vi "8step.vi"(6 "LINX Resource in":T1, 7 "Angle in":i32, 8 "error in (no error)":errorcluster, 9 "DO Channels":u8[](array[numeric]), 10 "CCW":bool, 11 "OK Button":bool) -> (0 "error out":errorcluster, 2 "LINX Resource out":T1, 3 "Actual angle out":dbl)   [LabVIEW 2020]
uses:
  <vilib>/MakerHub/LINX/Private/Type Defs/LINX Ref.ctl
  <vilib>/MakerHub/LINX/Private/Type Defs/Platform.ctl
  <vilib>/MakerHub/LINX/Private/Type Defs/Interface.ctl
  <vilib>/MakerHub/LINX/Private/Device/Type Defs/LINX Device Config.ctl
  <vilib>/MakerHub/LINX/Private/Device/Type Defs/TCP Config.ctl
  <vilib>/MakerHub/LINX/Private/Device/Type Defs/Channels.ctl
  <vilib>/MakerHub/LINX/Public/Peripherals/Digital/Digital Write N Chans.vi
  <vilib>/MakerHub/LINX/Private/Local IO/LinxDigitalWrite.vi
  <vilib>/MakerHub/LINX/Public/Utilities/Check Channel.vi
  <vilib>/MakerHub/LINX/Private/Utilties/Generate Error.vi
  <vilib>/MakerHub/LINX/LMH-LINX.lvlib
  <vilib>/MakerHub/LINX/Private/Device/Device.lvlib
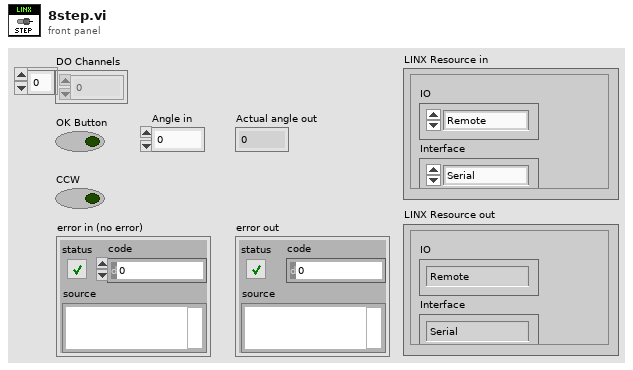
[diagram p1: front panel]
types:
  T1 = typedef "LMH-LINX.lvlib/LINX Ref.ctl" = cluster{"IO":T2, "Interface":T3, "LINX Device Config":T4}
  T2 = typedef "LMH-LINX.lvlib/Platform.ctl" = enum16{"Remote", "Local"}
  T3 = typedef "LMH-LINX.lvlib/Interface.ctl" = enum16{"Serial", "TCP"}
  T4 = typedef "LMH-LINX.lvlib/Device.lvlib/LINX Device Config.ctl" = cluster{"Interface":T3, "COM Port":refnum<visa-resource-name>, "TCP Configuration":T5, "Device Family":u8, "Device ID":u8, "Device Name":string, "TCP Ref":refnum<k5>, "Channels":T6}
  T5 = typedef "LMH-LINX.lvlib/Device.lvlib/TCP Config.ctl" = cluster{"IP Address":string, "Port":u16}
  T6 = typedef "LMH-LINX.lvlib/Channels.ctl" = cluster{"DI":u8[], "DO":u8[], "AI":u8[], "AO":u8[], "PWM":u8[], "QE":u8[], "UART":u8[], "I2C 2":u8[], "SPI":u8[], "CAN":u8[], "Servo":u8[], "AI Ref (V)":dbl, "AI Resolution (Bits)":u8, "AO Ref (V)":dbl, "AO Resolution (Bits)":u8}
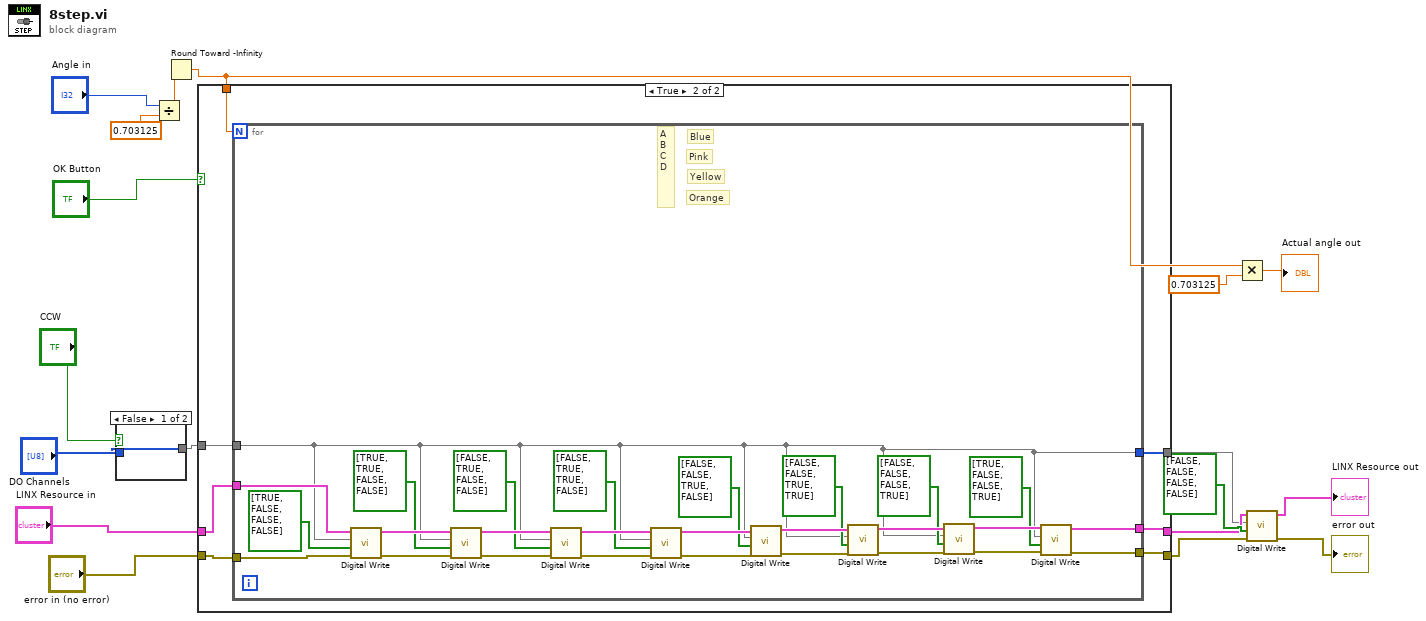
[diagram p0: block diagram]
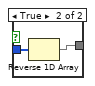
[diagram p2: hidden frame]
diagram:
  n1 = case shown="False" "CCW" {
    tunnel: "DO Channels" -> [w19 w21]
    tunnel: [w19 w20] -> w17
    frame False {
    }
    frame True {
      n2 = Reverse 1D Array(array=w21) -> (reversed array=w20:u8[])
    }
  }
  n3 = Divide(x="Angle in", y=0.703125) -> (x/y=w12:dbl)
  n4 = Round Toward -Infinity(1:w12) -> (0:w14:dbl)
  n5 = case shown="True" "OK Button" {
    tunnel: "LINX Resource in" -> [w24 w30]
    tunnel: [w24 w29] -> w7
    tunnel: "error in (no error)" -> [w23 w28]
    tunnel: [w23 w27] -> w9
    tunnel: w17 -> [w22 w31]
    tunnel: [w22 w26] -> w6
    tunnel: w14 -> [_ w25]
    frame False {
    }
    frame True {
      n6 = for {
        N: w25 -> [_]
        tunnel: w31 -> [w32]
        tunnel: w30 -> [w36]
        tunnel: [w35] -> w29
        tunnel: w28 -> [w34]
        tunnel: [w33] -> w27
        tunnel: [w32] -> w26
        # "A\nB\nC\nD"
        # "Orange"
        # "Yellow"
        # "Pink"
        # "Blue"
        n7 = call-poly <vilib>:"Digital Write.vi"("Error In"=w34, "Values"=bool[] [TRUE, FALSE, FALSE, FALSE], "DO Channels"=w32, "LINX Resource"=w36) -> ("Error Out"=w55:errorcluster, "LINX Resource"=w58:T1)  [unwired: 6 in]
        n8 = call-poly <vilib>:"Digital Write.vi"("Error In"=w55, "Values"=bool[] [TRUE, TRUE, FALSE, FALSE], "DO Channels"=w32, "LINX Resource"=w58) -> ("Error Out"=w54:errorcluster, "LINX Resource"=w57:T1)  [unwired: 6 in]
        n9 = call-poly <vilib>:"Digital Write.vi"("Error In"=w54, "Values"=bool[] [FALSE, TRUE, FALSE, FALSE], "DO Channels"=w32, "LINX Resource"=w57) -> ("Error Out"=w53:errorcluster, "LINX Resource"=w56:T1)  [unwired: 6 in]
        n10 = call-poly <vilib>:"Digital Write.vi"("Error In"=w53, "Values"=bool[] [FALSE, TRUE, TRUE, FALSE], "DO Channels"=w32, "LINX Resource"=w56) -> ("Error Out"=w44:errorcluster, "LINX Resource"=w48:T1)  [unwired: 6 in]
        n11 = call-poly <vilib>:"Digital Write.vi"("Error In"=w44, "Values"=bool[] [FALSE, FALSE, TRUE, FALSE], "DO Channels"=w32, "LINX Resource"=w48) -> ("Error Out"=w43:errorcluster, "LINX Resource"=w47:T1)  [unwired: 6 in]
        n12 = call-poly <vilib>:"Digital Write.vi"("Error In"=w43, "Values"=bool[] [FALSE, FALSE, TRUE, TRUE], "DO Channels"=w32, "LINX Resource"=w47) -> ("Error Out"=w42:errorcluster, "LINX Resource"=w46:T1)  [unwired: 6 in]
        n13 = call-poly <vilib>:"Digital Write.vi"("Error In"=w42, "Values"=bool[] [FALSE, FALSE, FALSE, TRUE], "DO Channels"=w32, "LINX Resource"=w46) -> ("Error Out"=w41:errorcluster, "LINX Resource"=w45:T1)  [unwired: 6 in]
        n14 = call-poly <vilib>:"Digital Write.vi"("Error In"=w41, "Values"=bool[] [TRUE, FALSE, FALSE, TRUE], "DO Channels"=w32, "LINX Resource"=w45) -> ("Error Out"=w33:errorcluster, "LINX Resource"=w35:T1)  [unwired: 6 in]
      }
    }
  }
  n15 = Multiply(x=w14, y=0.703125) -> (x*y=→"Actual angle out":dbl)
  n16 = call-poly <vilib>:"Digital Write.vi"("Error In"=w9, "Values"=bool[] [FALSE, FALSE, FALSE, FALSE], "DO Channels"=w6, "LINX Resource"=w7) -> ("Error Out"=→"error out":errorcluster, "LINX Resource"=→"LINX Resource out":T1)  [unwired: 6 in]
